vi "UR3_model-testing.vi"() -> ()   [LabVIEW 2024]
uses:
  <vilib>/Analysis/Matrix/Datatypes/RealMatrix.ctl
  <vilib>/robotics/Kinematics/Link/Joint Type.ctl
  <vilib>/robotics/Kinematics/Analytical/Initialize Generic Serial Arm.vi
  <vilib>/robotics/Kinematics/Robot/Inverse Kinematics (Point).vi
  <vilib>/robotics/Kinematics/Generate Joint Trajectory (Int).vi
  <vilib>/robotics/Kinematics/Analytical/NI_Robotics_AnalyticKinematics.lvlib
  <vilib>/robotics/Kinematics/Robot/NI_Robotics_Serial Robot Arm.lvclass
  <vilib>/robotics/Kinematics/Link/NI_Robotics_Link.lvclass
  <vilib>/robotics/Kinematics/Plotting/NI_Robotics_3DKinematics.lvlib
  <vilib>/robotics/Kinematics/NI_Kinematics.lvlib
  <vilib>/Analysis/Matrix/NI_Matrix.lvlib
panel:
  out "forward kinematics":T1
  out "joint position trajectory":dbl[](array[numeric])
  out "joint positions":dbl[](array[numeric])
  out "Animation":refnum<vi>(3d-picture)
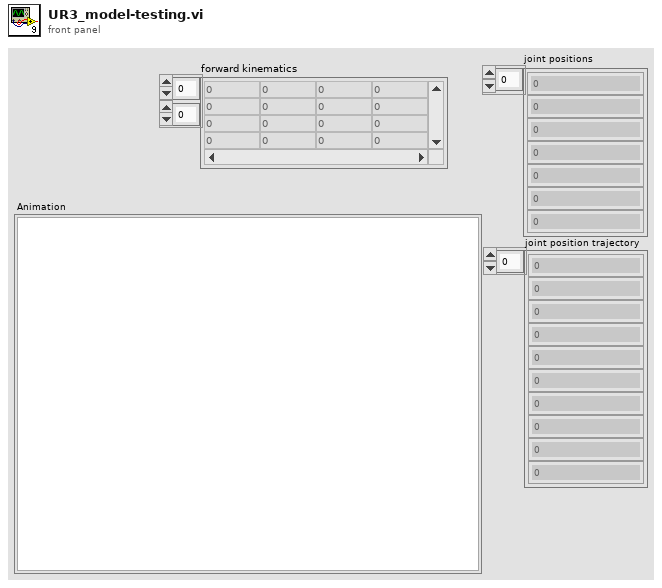
[diagram p1: front panel]
types:
  T1 = typedef "NI_Matrix.lvlib/RealMatrix.ctl" = dbl[][]
  T2 = typedef "NI_Robotics_Link.lvclass/Joint Type.ctl" = enum16{"Revolute", "Prismatic"}
  T3 = cluster{"alpha":dbl, "a":dbl, "theta":dbl, "d":dbl, "joint type":T2, " offset":dbl}[]
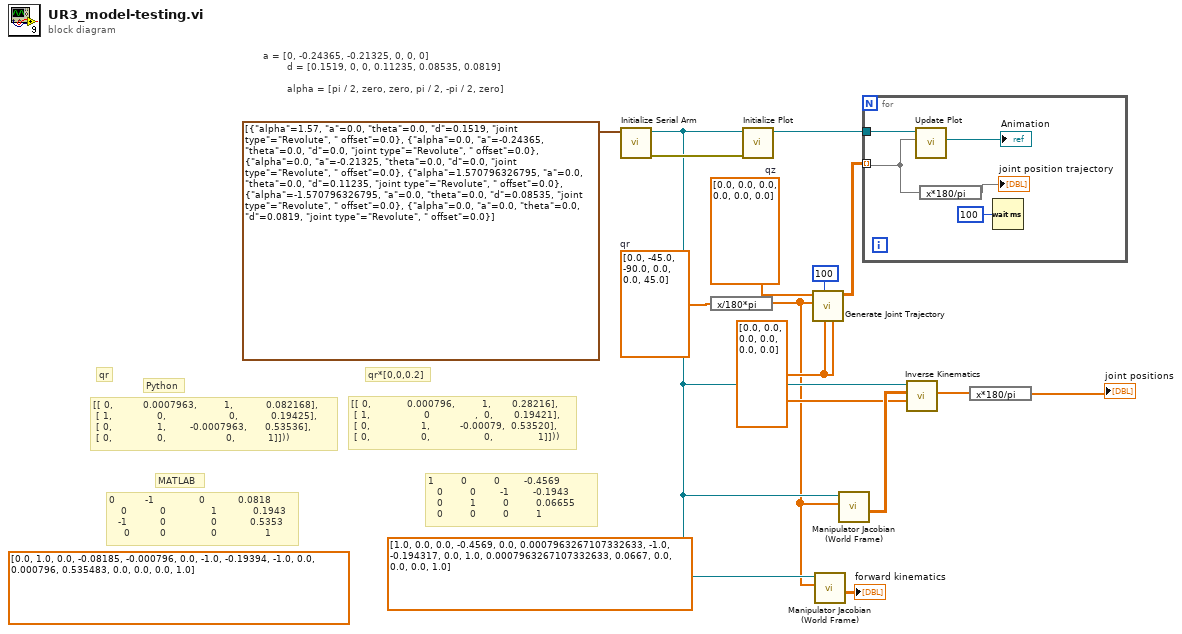
[diagram p0: block diagram]
diagram:
  (unwired) T1 [[1.0, 0.0, 0.0, -0.4569], [0.0, 0.0007963267107332633, -1.0, -0.194317], [0.0, 1.0, 0.0007963267107332633, 0.0667], [0.0, 0.0, 0.0, 1.0]] ("forward kinematics")
  (unwired) T1 [[0.0, 1.0, 0.0, -0.08185], [-0.000796, 0.0, -1.0, -0.19394], [-1.0, 0.0, 0.000796, 0.535483], [0.0, 0.0, 0.0, 1.0]] ("end effector transform")
  w2 = dbl[] [0.0, 0.0, 0.0, 0.0, 0.0, 0.0] ("start joint velocities")
  w11 = dbl[] [0.0, 0.0, 0.0, 0.0, 0.0, 0.0]  # qz
  w13 = dbl[] [0.0, -45.0, -90.0, 0.0, 0.0, 45.0]  # qr
  # "1         0         0        -0.4569    \n   0         0        -1        -0.1943    \n   0         1         0         0.06655   \n   0         0         0         1"
  # "a = [0, -0.24365, -0.21325, 0, 0, 0]\n        d = [0.1519, 0, 0, 0.11235, 0.08535, 0.0819]\n\n        alpha = [pi / 2, zero, zero, pi / 2, -pi / 2, zero]"
  # "qr*[0,0,0.2]"
  # "qr"
  # "[[ 0,          0.0007963,         1,           0.082168],\n [ 1,               0,                     0,           0.19425],\n [ 0,               1,        -0.0007963,      0.53536],\n [ 0,               0,                    0,           1]]))"
  # "MATLAB"
  # "0          -1               0           0.0818\n    0           0               1            0.1943\n   -1           0               0           0.5353\n     0          0               0                1"
  # "Python"
  # "[[ 0,            0.000796,         1,       0.28216],\n [ 1,                  0               ,  0,       0.19421],\n [ 0,                 1,          -0.00079,  0.53520],\n [ 0,                 0,                  0,               1]]))"
  n1 = call-poly <vilib>:"Initialize Serial Arm.vi"("kinematic parameters"=T3 [{"alpha"=1.57, "a"=0.0, "theta"=0.0, "d"=0.1519, "joint type"=enum."Revolute", " offset"=0.0}, {"alpha"=0.0, "a"=-0.24365, "theta"=0.0, "d"=0.0, "joint type"=enum."Revolute", " offset"=0.0}, {"alpha"=0.0, "a"=-0.21325, "theta"=0.0, "d"=0.0, "joint type"=enum."Revolute", " offset"=0.0}, {"alpha"=1.570796326795, "a"=0.0, "theta"=0.0, "d"=0.11235, "joint type"=enum."Revolute", " offset"=0.0}, {"alpha"=-1.570796326795, "a"=0.0, "theta"=0.0, "d"=0.08535, "joint type"=enum."Revolute", " offset"=0.0}, {"alpha"=0.0, "a"=0.0, "theta"=0.0, "d"=0.0819, "joint type"=enum."Revolute", " offset"=0.0}]) -> ("error out"=w12:errorcluster, "serial arm out"=w4:refnum<class "NI_Robotics_Serial Robot Arm.lvclass">)  [unwired: 9 in]
  n2 = expression code="x/180*pi"(w13) -> (w1:dbl[])
  n3 = call <vilib>:"Initialize Plot.vi"("error in (no error)"=w12, "serial arm in"=w4) -> ("serial arm out"=w8:refnum<class "NI_Robotics_Serial Robot Arm.lvclass">)  [unwired: 8 in, 1 out]
  n4 = call-poly <vilib>:"Generate Joint Trajectory.vi"("end joint velocities"=w2, "start joint velocities"=w2, "intermediate points"=100, "end joint positions"=w1, "start joint positions"=w11) -> ("joint position trajectory"=w10:dbl[][])  [unwired: 3 in, 3 out]
  n5 = call <vilib>:"Manipulator Jacobian (World Frame).vi"("joint positions"=w1, "serial arm in"=w4) -> ("forward kinematics"=→"forward kinematics":T1)  [unwired: 1 in, 8 out]
  n6 = call <vilib>:"Manipulator Jacobian (World Frame).vi"("joint positions"=w1, "serial arm in"=w4) -> ("forward kinematics"=w7:T1)  [unwired: 1 in, 8 out]
  n7 = for {
    tunnel: w10 -> [w16] mode=indexing
    tunnel: w8 -> [w18]
    n8 = call <vilib>:"Update Plot.vi"("joint positions"=w16, "serial arm in"=w18) -> ("serial arm scene"=→"Animation":refnum<vi>)  [unwired: 7 in, 2 out]
    n9 = expression code="x*180/pi"(w16) -> (→"joint position trajectory":dbl[])
    n10 = Wait (ms)(milliseconds to wait=u32 100) -> ()  [unwired: 1 out]
  }
  n11 = call-poly <vilib>:"Inverse Kinematics.vi"("current joint positions"=w2, "end effector transform"=w7, "serial arm in"=w4) -> ("joint positions"=w6:dbl[])  [unwired: 5 in, 3 out]
  n12 = expression code="x*180/pi"(w6) -> (→"joint positions":dbl[])
